vi "mod_Create Mask.vi"(0 "upper mask definition":cluster{"time":dbl, "power (dB)":dbl}[](array[cluster]) {"power (dB)" format="%.2f"; "time" format="%.2f"}, 5 "ideal profile definition":cluster{"time":dbl, "power (dB)":dbl}[](array[cluster]) {"power (dB)" format="%.2f"; "time" format="%.2f"}, 7 "lower mask definition":cluster{"time":dbl, "power (dB)":dbl}[](array[cluster]) {"power (dB)" format="%.2f"; "time" format="%.2f"}, 9 "dt":dbl=1.0 format="%.2p", 11 "interpolation":T1(ring)=enum."linear dB") -> (4 "upper mask":dbl[](array[numeric]) format="%.2f", 6 "ideal":dbl[](array[numeric]) format="%.2f", 8 "lower mask":dbl[](array[numeric]) format="%.2f")   [LabVIEW 2020, in "niDMT.lvlib"]
uses:
  <vilib>/addons/Modulation/niDMT.lvlib
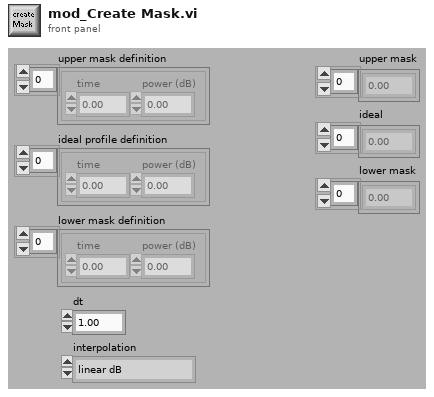
[diagram p1: front panel]
types:
  T1 = enum16{"linear power", "linear voltage", "linear dB"}
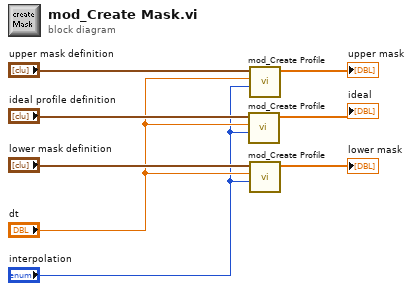
[diagram p0: block diagram]
diagram:
  n1 = call <vilib>:"mod_Create Profile.vi"("interpolation"="interpolation", "dt"="dt", "profile definition"="ideal profile definition") -> ("profile"=→"ideal":dbl[])  [unwired: 8 out]
  n2 = call <vilib>:"mod_Create Profile.vi"("interpolation"="interpolation", "dt"="dt", "profile definition"="upper mask definition") -> ("profile"=→"upper mask":dbl[])  [unwired: 8 out]
  n3 = call <vilib>:"mod_Create Profile.vi"("interpolation"="interpolation", "dt"="dt", "profile definition"="lower mask definition") -> ("profile"=→"lower mask":dbl[])  [unwired: 8 out]
